vi "NumberToArrayUint8.vi"(0 "Numeric 2":i16) -> (1 "Array":i8[](array[numeric]), 2 "Numeric":i32)   [LabVIEW 2011]
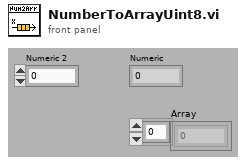
[diagram p1: front panel]
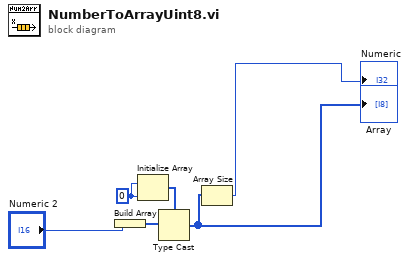
[diagram p0: block diagram]
diagram:
  w4 = i8 0 ("dimension size")
  n1 = Build Array("Numeric 2") -> (w2:i16[])
  n2 = Initialize Array(w4, w4) -> (w3:i8[])
  n3 = Type Cast(type=w3, x=w2) -> (*(type *) &x=w6:i8[])
  "Array" <- w6
  n4 = Array Size(array=w6) -> (size(s)=→"Numeric":i32)
